vi "StellarNetMath[Poly].vi"   [LabVIEW 2020]
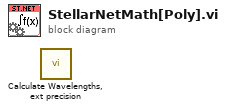
[diagram p0: block diagram]
diagram:
  n1 = call "Calculate Wavelengths, ext precision.vi"() -> ()  [unwired: 10 in, 2 out]
